vi "SubVI_Res_Table_data.vi"(7 "cmd":enum16{"ini", "write", "read"}(ring), 8 "error in (no error)":errorcluster caption="에러 입력(에러 없음)", 11 "Resister data":T1) -> (0 "error out":errorcluster caption="에러 출력", 3 "Result Table":T2)   [LabVIEW 2013]
uses:
  Ctrls/raw data type.ctl
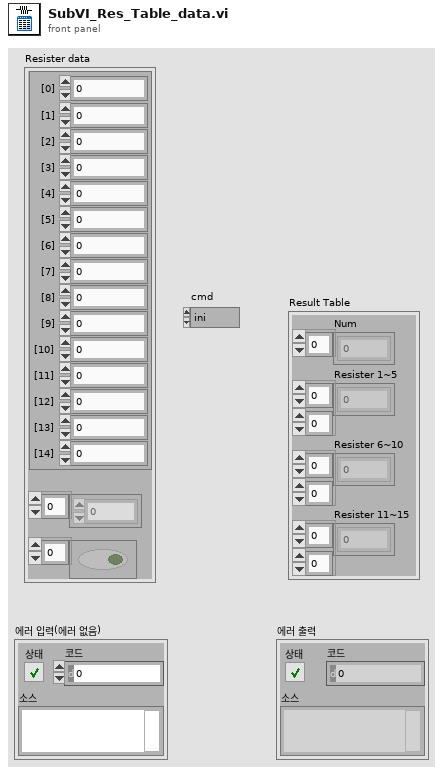
[diagram p1: front panel]
types:
  T1 = typedef "raw data type.ctl" = cluster{"Resistor values":cluster{"[0]":dbl, "[1]":dbl, "[2]":dbl, "[3]":dbl, "[4]":dbl, "[5]":dbl, "[6]":dbl, "[7]":dbl, "[8]":dbl, "[9]":dbl, "[10]":dbl, "[11]":dbl, "[12]":dbl, "[13]":dbl, "[14]":dbl}, "Resistor tables":u8[], "Pass Fails":bool[]}
  T2 = cluster{"Num":u32[], "Resister 1~5":u8[][], "Resister 6~10":u8[][], "Resister 11~15":u8[][]}
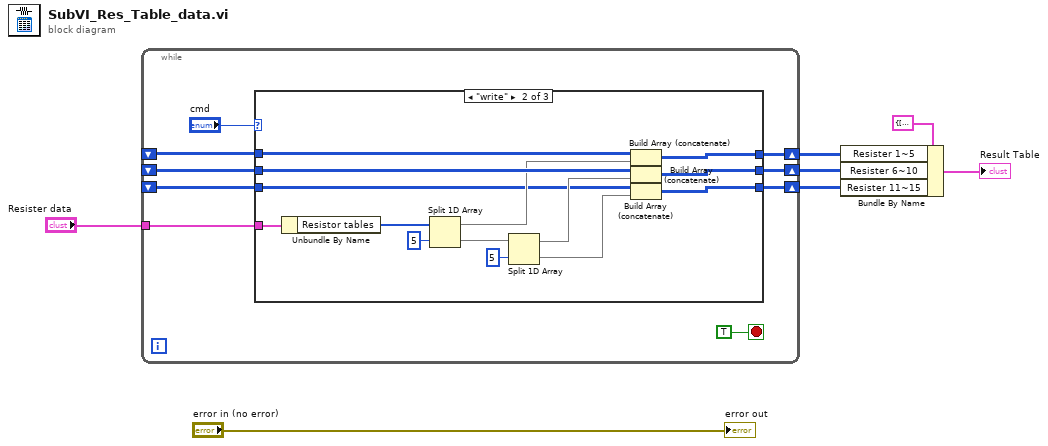
[diagram p0: block diagram]
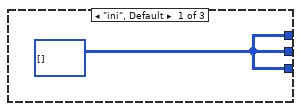
[diagram p2: hidden frame]
diagram:
  n1 = while {
    shift-right: [w14] -> w3
    shift-left: _ -> [w13]
    shift-right: [w12] -> w4
    shift-left: _ -> [w9]
    shift-right: [w11] -> w5
    shift-left: _ -> [w10]
    tunnel: "Resister data" -> [w8]
    stop <- TRUE stop-if-true
    n2 = case shown="\"write\"" "cmd" {
      tunnel: [w17 w20 w34] -> w14
      tunnel: w13 -> [_ w22 w34]
      tunnel: [w17 w21 w33] -> w12
      tunnel: [w17 w27 w32] -> w11
      tunnel: w10 -> [_ w28 w32]
      tunnel: w9 -> [_ w26 w33]
      tunnel: w8 -> [_ w18 _]
      frame "ini", Default {
        w17 = u8[][] [] ("Result Table data")
      }
      frame "write" {
        n3 = Unbundle By Name(w18) -> ("Resistor tables"=w19:u8[])
        n4 = Split 1D Array(array=w19, index=5 ("인덱스")) -> (first subarray=w25:u8[], second subarray=w31:u8[])
        n5 = Split 1D Array(array=w31, index=5 ("인덱스")) -> (first subarray=w24:u8[], second subarray=w23:u8[])
        n6 = Build Array (concatenate)(w28, w25) -> (w27:u8[][])
        n7 = Build Array (concatenate)(w26, w24) -> (w21:u8[][])
        n8 = Build Array (concatenate)(w22, w23) -> (w20:u8[][])
      }
      frame "read" {
      }
    }
  }
  n9 = Bundle By Name(cluster=T2 {"Num"=[1, 2, 3, 4, 5, 6, 7, 8, 9, 10, 11, 12, 13, 14, 15, 16, 17, 18, 19, 20, 21, 22, 23, 24, 25, 26, 27, 28, 29, 30, 31, 32, 33, 34, 35, 36, 37, 38, 39, 40, 41, 42, 43, 44, 45, 46, 47, 48, 49, 50, 51, 52, 53, 54, 55, 56, 57, 58, 59, 60, 61, 62, 63, 64, 65, 66, 67, 68, 69, 70, 71, 72, 73, 74, 75, 76, 77, 78, 79, 80, 81, 82, 83, 84, 85, 86, 87, 88, 89, 90, 91, 92, 93, 94, 95, 96, 97, 98, 99, 100], "Resister 1~5"=[[1, 1, 1, 0, 0], [1, 1, 1, 0, 0], [1, 1, 1, 0, 0], [1, 1, 1, 0, 0], [1, 1, 1, 0, 0], [1, 1, 1, 0, 0], [1, 1, 1, 0, 0], [1, 1, 1, 0, 0], [1, 1, 1, 0, 0], [1, 1, 1, 0, 0]], "Resister 6~10"=[[1, 1, 1, 1, 0], [1, 1, 1, 1, 0], [1, 1, 1, 1, 0], [1, 1, 1, 1, 0], [1, 1, 1, 1, 0], [1, 1, 1, 1, 0], [1, 1, 1, 1, 0], [1, 1, 1, 1, 0], [1, 1, 1, 1, 0], [1, 1, 1, 1, 0]], "Resister 11~15"=[[0, 0, 1, 1, 1], [0, 0, 1, 1, 1], [0, 0, 1, 1, 1], [0, 0, 1, 1, 1], [0, 0, 1, 1, 1], [0, 0, 1, 1, 1], [0, 0, 1, 1, 1], [0, 0, 1, 1, 1], [0, 0, 1, 1, 1], [0, 0, 1, 1, 1]]} ("Result Table"), "Resister 1~5"=w5, "Resister 6~10"=w4, "Resister 11~15"=w3) -> (→"Result Table":T2)
  "error out" <- "error in (no error)"
